vi "GetModuleCentre (SubVI).vi"(3 "error in (no error)":errorcluster, 4 "4x3 Array of Fiducial Coordinates":dbl[][](array[numeric])) -> (0 "error out":errorcluster, 1 "y, centre":dbl, 2 "x, centre":dbl)   [LabVIEW 2017]
panel:
  # "Taking in an array of the coordinates (x, y, z) of the\nfour fiducial marks on a module, entred in the array in the order \ncorner A, B, C, and D, this SubVI returns the x and y coordinates \nof the centre of the module."
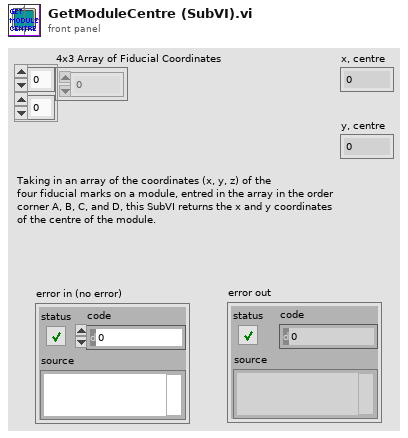
[diagram p1: front panel]
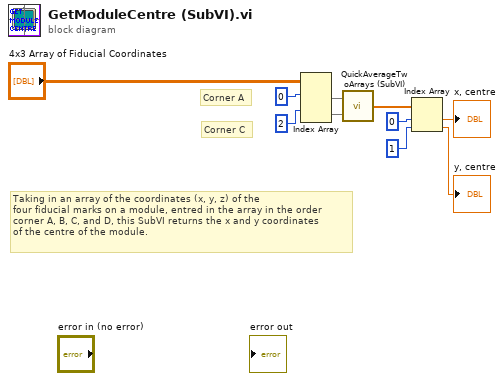
[diagram p0: block diagram]
diagram:
  # "Taking in an array of the coordinates (x, y, z) of the\nfour fiducial marks on a module, entred in the array in the order \ncorner A, B, C, and D, this SubVI returns the x and y coordinates \nof the centre of the module."
  # "Corner C"
  # "Corner A"
  n1 = Index Array(array="4x3 Array of Fiducial Coordinates", index (row) #1=0 ("index (row)"), index (row) #2=2 ("disabled index (row)")) -> (element #1=w3:dbl[], element #2=w4:dbl[])  [unwired: 2 in]
  n2 = call "QuickAverageTwoArrays (SubVI).vi"("B"=w4, "A"=w3) -> ("Average of A and B"=w5:dbl[])
  n3 = Index Array(array=w5, index #1=0 ("index"), index #2=1 ("index")) -> (element #1=→"x, centre":dbl, element #2=→"y, centre":dbl)
